vi "loadMapping.vi"(8 "error in (no error)":errorcluster, 9 "Channel.lvclass":refnum<class "Channel.lvclass">, 10 "xmlNode.lvclass":refnum<class "xmlNode.lvclass">, 11 "deviceDataBase in":refnum<class "deviceDataBase.lvclass">) -> (0 "error out":errorcluster, 1 "Channel.lvclass out":refnum<class "Channel.lvclass">, 2 "xmlNode out":refnum<class "xmlNode.lvclass">, 3 "deviceDataBase out":refnum<class "deviceDataBase.lvclass">)   [LabVIEW 2011, in "Tools.lvlib" / "DatabaseHelpers.lvlib" / "deviceDataBase.lvclass"]
uses:
  deviceDataBase.lvclass
  xmlNode/xmlNode.lvclass
  Database Objects/Channel/Channel.lvclass
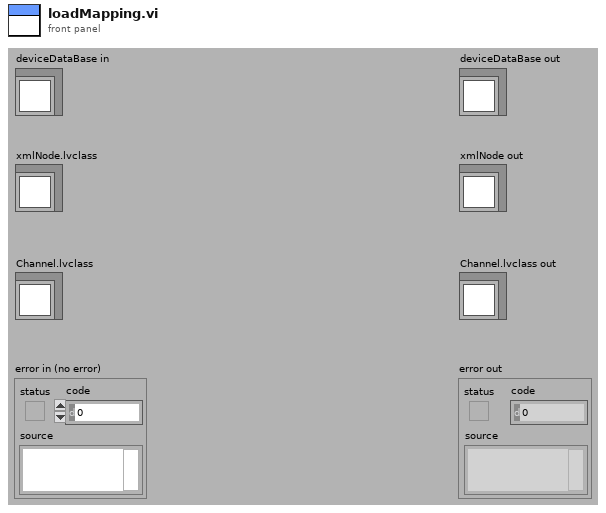
[diagram p1: front panel]
types:
  T1 = cluster{"attribute string":string, "stringValue":string}
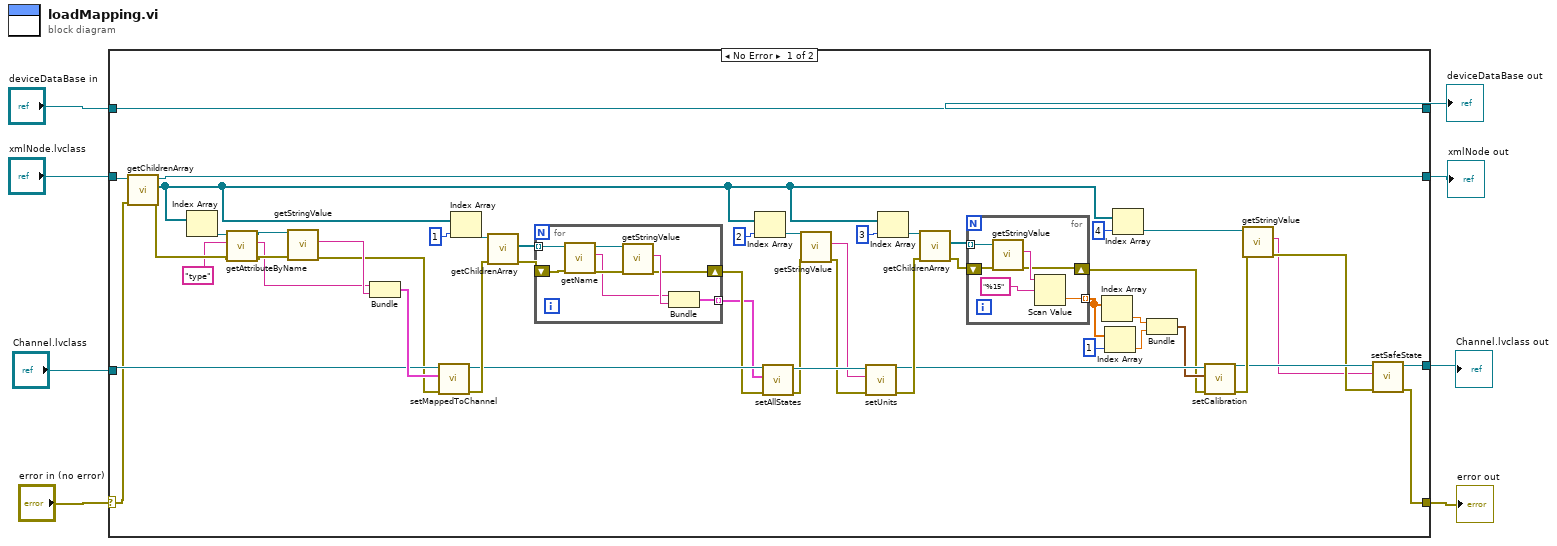
[diagram p0: block diagram]
diagram:
  n1 = case shown="No Error" "error in (no error)" {
    selector: "error in (no error)" -> [w16 w73]
    tunnel: [w19 w73] -> w7
    tunnel: [w57 w72] -> w5
    tunnel: "deviceDataBase in" -> [w57 w72]
    tunnel: "xmlNode.lvclass" -> [w56 _]
    tunnel: "Channel.lvclass" -> [w53 _]
    tunnel: [w18 _] -> w2
    tunnel: [w17 _] -> w1
    frame No Error {
      n2 = call-dynamic "getChildrenArray.vi"("error in (no error)"=w16, "xmlNode.lvclass in"=w56) -> ("error out"=w15:errorcluster, "Children"=w26:refnum<class "xmlNode.lvclass">[], "xmlNode.lvclass out"=w17:refnum<class "xmlNode.lvclass">)  [unwired: 7 in]
      n3 = Index Array(array=w26) -> (element=w14:refnum<class "xmlNode.lvclass">)  [unwired: 1 in]
      n4 = call-dynamic "getAttributeByName.vi"("error in (no error)"=w15, "AttributeName"="type", "xmlNode in"=w14) -> ("error out"=w12:errorcluster, "attribute string"=w11:string, "xmlNode out"=w13:refnum<class "xmlNode.lvclass">)  [unwired: 6 in]
      n5 = call-dynamic "getStringValue.vi"("error in (no error)"=w12, "xmlNode.lvclass in"=w13) -> ("error out"=w52:errorcluster, "stringValue"=w55:string)  [unwired: 7 in, 1 out]
      n6 = Bundle("attribute string"=w11, "stringValue"=w55) -> (w54:T1)  [unwired: 1 in]
      n7 = call "setMappedToChannel.vi"("error in (no error)"=w52, "mappedTo"=w54, "Channel.lvclass in"=w53) -> ("error out"=w49:errorcluster, "Channel.lvclass out"=w46:refnum<class "Channel.lvclass">)  [unwired: 7 in]
      n8 = Index Array(array=w26, index=1) -> (element=w50:refnum<class "xmlNode.lvclass">)
      n9 = call-dynamic "getChildrenArray.vi"("error in (no error)"=w49, "xmlNode.lvclass in"=w50) -> ("error out"=w47:errorcluster, "Children"=w48:refnum<class "xmlNode.lvclass">[])  [unwired: 7 in, 1 out]
      n10 = for {
        shift-right: [w65] -> w45
        shift-left: w47 -> [w68]
        tunnel: w48 -> [w71] mode=indexing
        tunnel: [w66] -> w21 mode=indexing
        n11 = call-dynamic "getName.vi"("error in (no error)"=w68, "xmlNode.lvclass in"=w71) -> ("error out"=w69:errorcluster, "name"=w64:string, "xmlNode.lvclass out"=w70:refnum<class "xmlNode.lvclass">)  [unwired: 7 in]
        n12 = call-dynamic "getStringValue.vi"("error in (no error)"=w69, "xmlNode.lvclass in"=w70) -> ("error out"=w65:errorcluster, "stringValue"=w67:string)  [unwired: 7 in, 1 out]
        n13 = Bundle("name"=w64, "stringValue"=w67) -> (w66:cluster{"name":string, "stringValue":string})  [unwired: 1 in]
      }
      n14 = Index Array(array=w26, index=2) -> (element=w42:refnum<class "xmlNode.lvclass">)
      n15 = call "setAllStates.vi"("error in (no error)"=w45, "states"=w21, "Channel.lvclass in"=w46) -> ("error out"=w41:errorcluster, "Channel.lvclass out"=w43:refnum<class "Channel.lvclass">)  [unwired: 7 in]
      n16 = call-dynamic "getStringValue.vi"("error in (no error)"=w41, "xmlNode.lvclass in"=w42) -> ("error out"=w40:errorcluster, "stringValue"=w39:string)  [unwired: 7 in, 1 out]
      n17 = call-dynamic "setUnits.vi"("error in (no error)"=w40, "units"=w39, "Channel.lvclass in"=w43) -> ("error out"=w36:errorcluster, "Channel.lvclass out"=w31:refnum<class "Channel.lvclass">)  [unwired: 7 in]
      n18 = Index Array(array=w26, index=3) -> (element=w37:refnum<class "xmlNode.lvclass">)
      n19 = call-dynamic "getChildrenArray.vi"("error in (no error)"=w36, "xmlNode.lvclass in"=w37) -> ("error out"=w34:errorcluster, "Children"=w35:refnum<class "xmlNode.lvclass">[])  [unwired: 7 in, 1 out]
      n20 = for {
        tunnel: w35 -> [w63] mode=indexing
        tunnel: [w59] -> w33 mode=indexing
        shift-right: [w58] -> w27
        shift-left: w34 -> [w62]
        n21 = call-dynamic "getStringValue.vi"("error in (no error)"=w62, "xmlNode.lvclass in"=w63) -> ("error out"=w58:errorcluster, "stringValue"=w61:string)  [unwired: 7 in, 1 out]
        n22 = Scan Value(string=w61, format string="%15") -> (value=w59:dbl)  [unwired: 1 in, 1 out]
      }
      n23 = Index Array(array=w33) -> (element=w30:dbl)  [unwired: 1 in]
      n24 = Index Array(array=w33, index=1) -> (element=w29:dbl)
      n25 = Index Array(array=w26, index=4) -> (element=w24:refnum<class "xmlNode.lvclass">)
      n26 = Bundle(w30, w29) -> (w28:cluster{dbl, dbl})  [unwired: 1 in]
      n27 = call "setCalibration.vi"("error in (no error)"=w27, "calibration"=w28, "Channel.lvclass in"=w31) -> ("error out"=w23:errorcluster, "Channel.lvclass out"=w22:refnum<class "Channel.lvclass">)  [unwired: 7 in]
      n28 = call-dynamic "getStringValue.vi"("error in (no error)"=w23, "xmlNode.lvclass in"=w24) -> ("error out"=w20:errorcluster, "stringValue"=w9:string)  [unwired: 7 in, 1 out]
      n29 = call "setSafeState.vi"("error in (no error)"=w20, "safe_state"=w9, "Channel.lvclass in"=w22) -> ("error out"=w19:errorcluster, "Channel.lvclass out"=w18:refnum<class "Channel.lvclass">)  [unwired: 7 in]
    }
    frame Error {
    }
  }
  "error out" <- w7
  "deviceDataBase out" <- w5
  "xmlNode out" <- w1
  "Channel.lvclass out" <- w2
